vi "Set Cell Value  Range.vi"(4 "Excel._Worksheet":refnum<k7>, 5 "error in":errorcluster caption="错误输入（无错误）", 6 "Value":string caption="值", 7 "Col":i32 caption="列", 8 "Row":i32 caption="行") -> (0 "error out":errorcluster caption="错误输出", 1 "Cell":string caption="单元格", 2 "Range":refnum<k7> caption="范围", 3 "Excel._Worksheet":refnum<k7>)   [LabVIEW 2014]
doc: "本VI会将工作表中由“行：列”指定的单元格的值设置为输入“值”。首先将行和列的数值输入转换为Excel格式的A1和B1等，然后执行工作表对象的“范围方法”并设置范围的“值”属性。在循环的每次迭代中都将释放范围的自动化引用句柄。"
panel:
  in  "dummy Range":refnum<k7> caption="虚设范围"
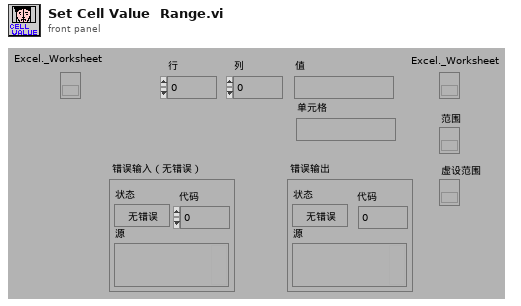
[diagram p1: front panel]
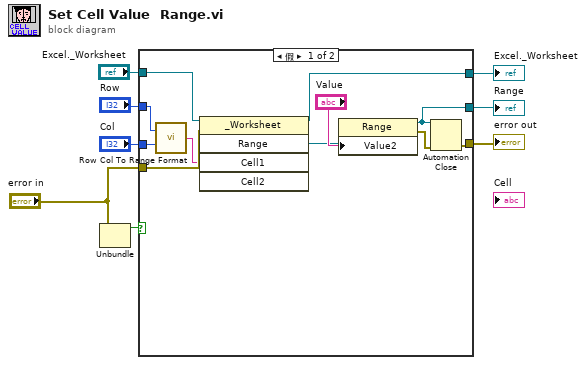
[diagram p0: block diagram]
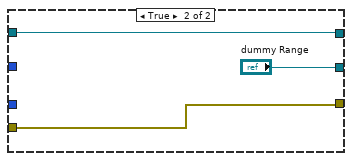
[diagram p2: hidden frame]
diagram:
  n1 = Unbundle("error in") -> ("status"=w4:bool)  [unwired: 2 out]
  n2 = case shown="假" w4 {
    tunnel: "Col" -> [w19 _]
    tunnel: "Row" -> [w18 _]
    tunnel: "error in" -> [w13 w22]
    tunnel: [w15 w22] -> w6
    tunnel: [w12 w21] -> w3
    tunnel: "Excel._Worksheet" -> [w11 w21]
    tunnel: [w14 "dummy Range"] -> w1
    frame False {
      n3 = call "Row Col To Range Format.vi"("Column"=w19, "Row"=w18) -> ("Output String"=w9:string)
      n4 = invoke class="_Worksheet" method="Range"(reference=w11, error in=w13, "Cell1"=w9) -> (reference out=w12:refnum<k7>, "Range"=w10:refnum<k7>)  [unwired: 2 in, 3 out]
      n5 = property class="Range"(reference=w10, "Value2"="Value") -> (reference out=w14:refnum<k7>, error out=w16:errorcluster)  [unwired: 1 in]
      n6 = Automation Close(3:w16, 5:w14) -> (0:w15:errorcluster)
    }
    frame True {
    }
  }
  "Excel._Worksheet" <- w3
  "error out" <- w6
  "Range" <- w1
